vi "HOL_Robot Global Data.vi"() -> ()   [LabVIEW 2019]
doc: "This global VI can contain as many global variables as you need. Place a control on the panel, give it a good name. To read or write to it from a VI, drag the icon to the diagram of that VI. You can also drag from the project. Click on the node to change which global you access. You shouldn't have multiple locations writing to a global or it will cause a race-condition."
uses:
  <vilib>/Rock Robotics/WPI/Camera/WPI_CameraImageSize.ctl
  <vilib>/Rock Robotics/WPI/DriverStation/WPI_DriverStationRobotMode2.ctl
panel:
  out "Traj Heading Dmd":dbl format="%17.2f"
  out "Traj Y Corr":dbl format="%17.2f"
  out "Traj X Corr":dbl format="%17.2f"
  out "Traj Closed Loop":bool
  out "Traj Curvature Sample":dbl format="%17.2f"
  out "Traj Velocity Sample":dbl format="%17.2f"
  out "Traj Heading Sample":dbl format="%17.2f"
  out "Traj Y Sample":dbl format="%17.2f"
  out "Traj X Sample":dbl format="%17.2f"
  out "Mod Swerve in Deadband":bool
  out "Mod Swerve On Targ":bool[](array[boolean])
  out "Mod Swerve Err":dbl[](array[numeric]) format="%17.3f"
  out "Mod Speed Err":dbl[](array[numeric]) format="%17.3f"
  out "Cont. Orientation Correct CO":dbl format="%17.3f"
  out "Cont. Orientation Angle Error":dbl format="%17.3f"
  out "Chassis vOmega Speed":dbl format="%17.3f"
  out "Chassis vY Speed":dbl format="%17.3f"
  out "Chassis vX Speed":dbl format="%17.3f"
  out "Mod Swerve Out":dbl[](array[numeric]) format="%17.3f"
  out "Mod Wheel Out":dbl[](array[numeric]) format="%17.3f"
  out "Mod Angle Act":dbl[](array[numeric]) format="%17.3f"
  out "Mod Speed Act":dbl[](array[numeric]) format="%17.3f"
  out "Mod Angle Dmd":dbl[](array[numeric]) format="%17.3f"
  out "Mod Speed Dmd":dbl[](array[numeric]) format="%17.3f"
  out "Chassis vOmega Dmd":dbl format="%17.3f"
  out "Chassis vY Dmd":dbl format="%17.3f"
  out "Chassis vX Dmd":dbl format="%17.3f"
  out "GyroHeading":dbl format="%17.2f"
  out "Cont. Orientation Angle Dmd":dbl format="%17.3f"
  out "Drv Omega Vel Dmd":dbl format="%17.3f"
  out "Drv Y Vel Dmd":dbl format="%17.3f"
  out "Drv X Vel Dmd":dbl format="%17.3f"
  out "Traj_IsGood":bool
  out "Traj_Total_Time":dbl format="%17.2f"
  out "Traj_Total_States":dbl format="%17.2f"
  out "Traj Heading Err":dbl format="%17.2f"
  out "Traj Y Err":dbl format="%17.2f"
  out "Traj X Err":dbl format="%17.2f"
  out "Traj_OnTarget":bool
  out "GyroCont":dbl format="%17.2f"
  out "DrvDistCalcLeft":dbl format="%17.2f"
  out "DrvDistCalcRight":dbl format="%17.2f"
  out "DrvDistReadLeft":dbl format="%17.2f"
  out "DrvDistReadRight":dbl format="%17.2f"
  out "DrvSpeedLeft":dbl format="%17.2f"
  out "DrvSpeedRight":dbl format="%17.2f"
  out "DrvMotorOutLeft":dbl format="%17.2f"
  out "DrvMotorOutRight":dbl format="%17.2f"
  out "DrvSpeedDmdLeft":dbl format="%17.2f"
  out "DrvSpeedDmdRight":dbl format="%17.2f"
  out "DrvSpeedTargLeft":dbl format="%17.2f"
  out "DrvSpeedTargRight":dbl format="%17.2f"
  in  "Robot Mode":T1
  in  "image size":T2=enum."320x240"
  in  "Enable Vision":bool
  # "Left over from diferential drive!!"
  # "swerve drive demands"
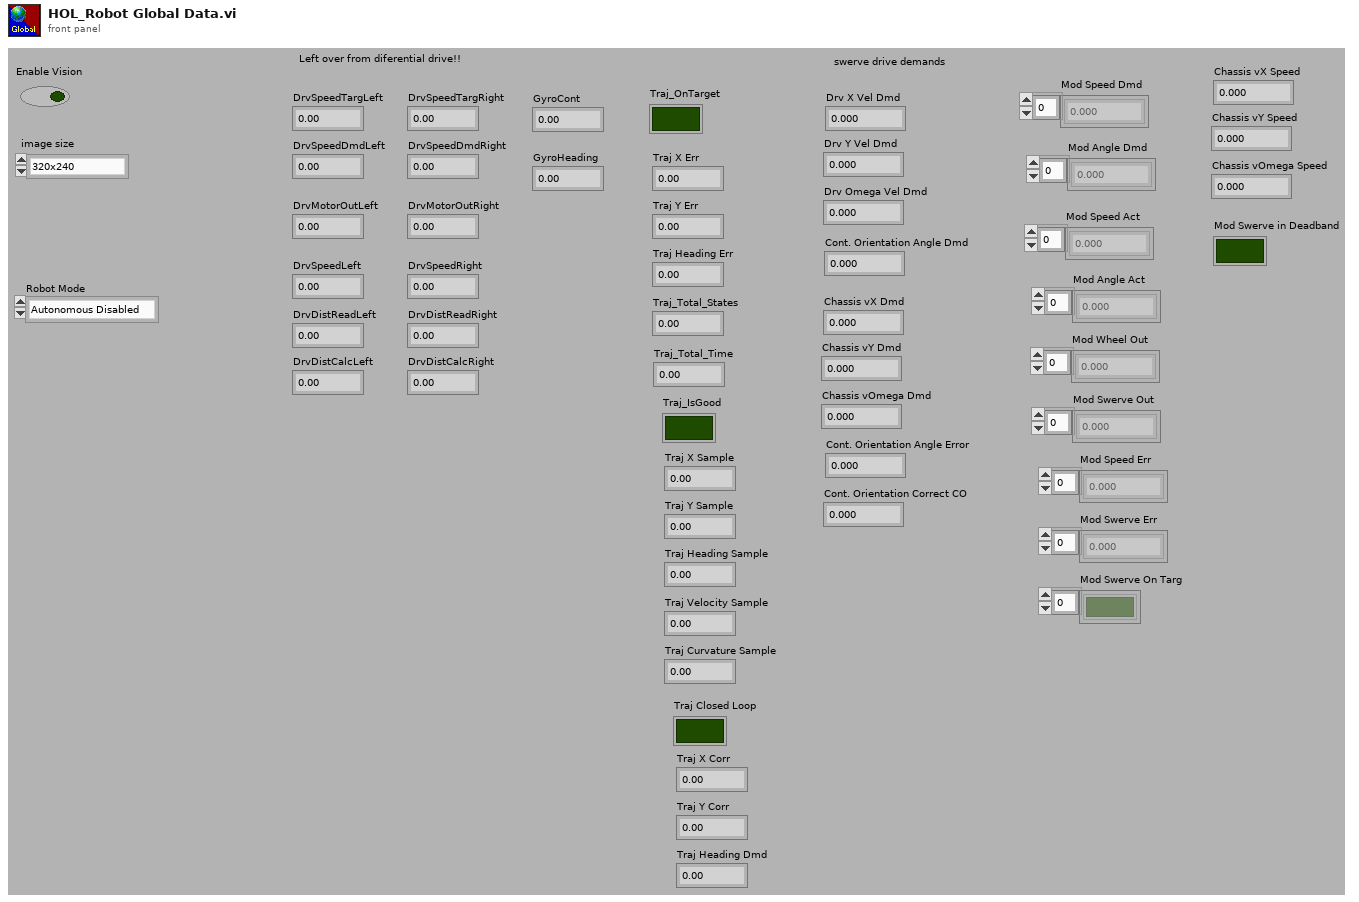
[diagram p1: front panel]
types:
  T1 = typedef "WPI_DriverStationRobotMode2.ctl" = enum16{"Autonomous Disabled", "Autonomous Enabled", "Teleop Disabled", "Teleop Enabled", "Disconnected", "Finish", "Test Disabled", "Test Enabled", "Emergency Stopped"}
  T2 = typedef "WPI_CameraImageSize.ctl" = enum16{"640x480", "320x240", "160x120", "Custom"}
diagram:
